vi "recIsCamRam.vi"(0 "Camera in":refnum<class "Camera.lvclass">, 11 "error in (no error)":errorcluster) -> (4 "Camera out":refnum<class "Camera.lvclass">, 6 "isCamram":bool, 15 "error out":errorcluster)   [LabVIEW 2019, in "Camera.lvclass"]
doc: "Determines if the current recorder mode uses internal camera RAM (CAMRAM)"
uses:
  Camera.lvclass
  Camera.lvclass/Camera.ctl
  pco.recorder/Recorder.lvlib
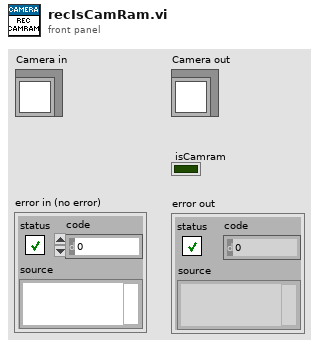
[diagram p1: front panel]
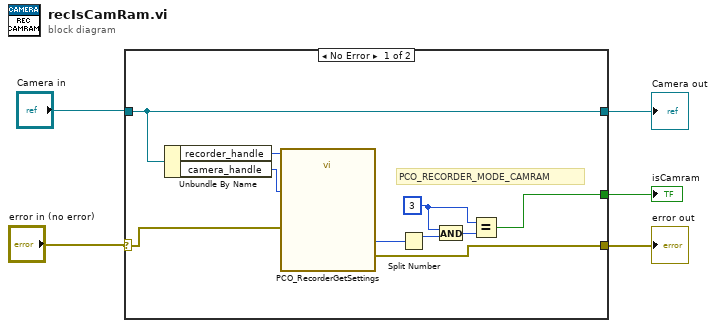
[diagram p0: block diagram]
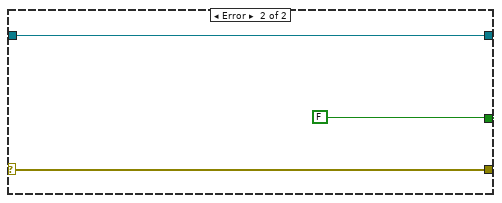
[diagram p2: hidden frame]
diagram:
  n1 = case shown="No Error" "error in (no error)" {
    selector: "error in (no error)" -> [w13 w18]
    tunnel: [w6 w18] -> w3
    tunnel: [w15 w17] -> w4
    tunnel: "Camera in" -> [w15 w17]
    tunnel: [w7 FALSE] -> w1
    frame No Error {
      w8 = u16 3
      # "PCO_RECORDER_MODE_CAMRAM"
      n2 = Unbundle By Name(w15) -> ("recorder_handle"=w14:u64, "camera_handle"=w12:u64)
      n3 = call "PCO_RecorderGetSettings.vi"("phRec"=w14, "phCam"=w12, "error in (no error)"=w13) -> ("dwRecMode"=w11:u32, "error out"=w6:errorcluster)  [unwired: 4 in, 7 out]
      n4 = Split Number(x=w11) -> (hi(x)=w10:u16)  [unwired: 1 out]
      n5 = And(x=w8, y=w10) -> (x .and. y?=w9:u16)
      n6 = Equal?(x=w8, y=w9) -> (x = y?=w7:bool)
    }
    frame Error {
    }
  }
  "error out" <- w3
  "Camera out" <- w4
  "isCamram" <- w1
